vi "Ensure Visible.vi"(10 "Line Numbers":refnum<vi>, 11 "String in":refnum<vi>) -> (2 "Scroll Position":u32, 3 "String out":refnum<vi>)   [LabVIEW 2016, in "Code String.lvclass"]
doc: "Checks the scroll position of <b>String</b> against the selected line in <b>Line Numbers</b> and adjusts the scroll position if the selected line is not range.\nReturns the resulting <b>Scroll Position</b>.\n--------------------\nCopyright (c) 2019 Analog Devices, Inc. All rights reserved.\n\nRedistribution and use in source and binary forms, with or without modification,\nare permitted provided that the following conditions are met:\n - Redistributions of source code must retain the above copyright notice, this\n list of conditions and the following disclaimer.\n - Redistributions in binary form must reproduce the above copyright notice,\n this list of conditions and the following disclaimer in the documentation\n and/or other materials provided with the distribution.\n - Modified versions of the software must be conspicuously marked as such.\n - This software is licensed solely and exclusively for use with\n processors/products manufactured by or for Analog Devices, Inc.\n - This software may not be combined or merged with other code in any manner\n that would cause the software to become subject to terms and conditions\n which differ from those listed here.\n - Neither the name of Analog Devices, Inc. nor the names of its contributors\n may be used to endorse or promote products derived from this software\n without specific prior written permission.\n - The use of this software may or may not infringe the patent rights of one or\n more patent holders. This license does not release you from the requirement\n that you obtain separate licenses from these patent holders to use this\n software.\n\nTHIS SOFTWARE IS PROVIDED BY ANALOG DEVICES, INC. AND CONTRIBUTORS \"AS IS\" AND\nANY EXPRESS OR IMPLIED WARRANTIES, INCLUDING, BUT NOT LIMITED TO,\nNON-INFRINGEMENT, TITLE, MERCHANTABILITY AND FITNESS FOR A PARTICULAR PURPOSE\nARE DISCLAIMED. IN NO EVENT SHALL ANALOG DEVICES, INC. OR CONTRIBUTORS BE LIABLE\nFOR ANY DIRECT, INDIRECT, INCIDENTAL, SPECIAL, EXEMPLARY, PUNITIVE OR\nCONSEQUENTIAL DAMAGES (INCLUDING, BUT NOT LIMITED TO, DAMAGES ARISING OUT OF\nCLAIMS OF INTELLECTUAL PROPERTY RIGHTS INFRINGEMENT; PROCUREMENT OF SUBSTITUTE\nGOODS OR SERVICES; LOSS OF USE, DATA, OR PROFITS; OR BUSINESS INTERRUPTION)\nHOWEVER CAUSED AND ON ANY THEORY OF LIABILITY, WHETHER IN CONTRACT, STRICT\nLIABILITY, OR TORT (INCLUDING NEGLIGENCE OR OTHERWISE) ARISING IN ANY WAY OUT OF\nTHE USE OF THIS SOFTWARE, EVEN IF ADVISED OF THE POSSIBILITY OF SUCH DAMAGE.\n\n2019-01-10-7CBSD SLA"
uses:
  Code String.lvclass
panel:
  # "Copyright (c) 2019 Analog Devices, Inc.  All rights reserved.\n\nRedistribution and use in source and binary forms, with or without modification,\nare permitted provided that the following conditions are met:\n  - Redistributions of source code must retain the above copyright notice, this\n    list of conditions and the following disclaimer.\n  - Redistributions in binary form must reproduce the above copyright notice,\n    this list of conditions and the following disclaimer in the documentation\n    and/or other materials provided with the distribution.\n  - Modified versions of the software must be conspicuously marked as such.\n  - This software is licensed solely and exclusively for use with\n    processors/products manufactured by or for Analog Devices, Inc.\n  - This software may not be combined or merged with other code in any manner\n    that would cause the software to become subject to terms and conditions\n    which differ from those listed here.\n  - Neither the name of Analog Devices, Inc. nor the names of its contributors\n    may be used to endorse or promote products derived from this software\n    without specific prior written permission.\n  - The use of this software may or may not infringe the patent rights of one or\n    more patent holders.  This license does not release you from the requirement\n    that you obtain separate licenses from these patent holders to use this\n    software.\n\nTHIS SOFTWARE IS PROVIDED BY ANALOG DEVICES, INC. AND CONTRIBUTORS \"AS IS\" AND\nANY EXPRESS OR IMPLIED WARRANTIES, INCLUDING, BUT NOT LIMITED TO,\nNON-INFRINGEMENT, TITLE, MERCHANTABILITY AND FITNESS FOR A PARTICULAR PURPOSE\nARE DISCLAIMED. IN NO EVENT SHALL ANALOG DEVICES, INC. OR CONTRIBUTORS BE LIABLE\nFOR ANY DIRECT, INDIRECT, INCIDENTAL, SPECIAL, EXEMPLARY, PUNITIVE OR\nCONSEQUENTIAL DAMAGES (INCLUDING, BUT NOT LIMITED TO, DAMAGES ARISING OUT OF\nCLAIMS OF INTELLECTUAL PROPERTY RIGHTS INFRINGEMENT; PROCUREMENT OF SUBSTITUTE\nGOODS OR SERVICES; LOSS OF USE, DATA, OR PROFITS; OR BUSINESS INTERRUPTION)\nHOWEVER CAUSED AND ON ANY THEORY OF LIABILITY, WHETHER IN CONTRACT, STRICT\nLIABILITY, OR TORT (INCLUDING NEGLIGENCE OR OTHERWISE) ARISING IN ANY WAY OUT OF\nTHE USE OF THIS SOFTWARE, EVEN IF ADVISED OF THE POSSIBILITY OF SUCH DAMAGE.\n\n2019-01-10-7CBSD SLA"
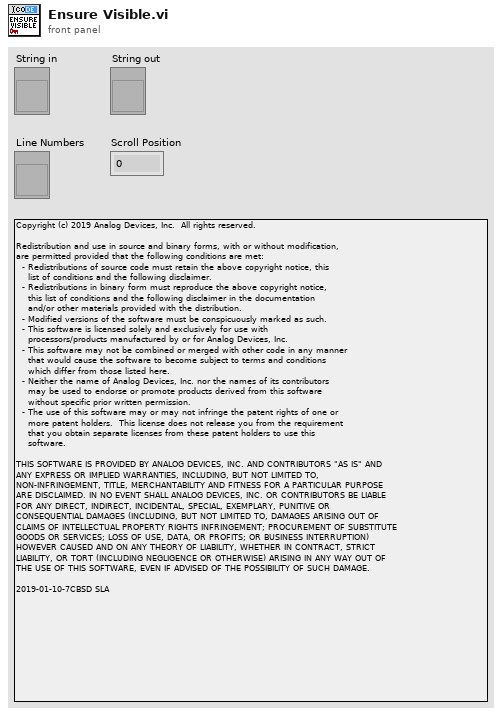
[diagram p1: front panel]
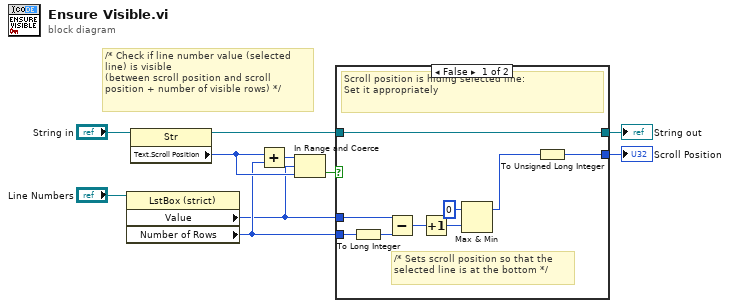
[diagram p0: block diagram]
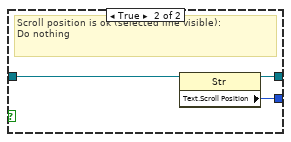
[diagram p2: hidden frame]
diagram:
  # "/* Check if line number value (selected line) is visible\n(between scroll position and scroll position + number of visible rows) */"
  n1 = property on="Property Node" class="LstBox (strict)"(reference="Line Numbers") -> ("Value"=w1:i32, "Number of Rows"=w2:u32)  [unwired: 1 in, 2 out]
  n2 = property on="Property Node" class="Str"(reference="String in") -> (reference out=w5:refnum<vi>, "Text.Scroll Position"=w6:u32)  [unwired: 1 in, 1 out]
  n3 = Add(x=w6, y=w2) -> (x+y=w7:u32)
  n4 = In Range and Coerce(upper limit=w7, x=w1, lower limit=w6) -> (In Range?=w4:bool)  [unwired: 1 out]
  n5 = case shown="False" w4 {
    tunnel: w5 -> [w19 w22]
    tunnel: [w11 w21] -> w8
    tunnel: [w19 w20] -> w3
    tunnel: w2 -> [w15 _]
    tunnel: w1 -> [w14 _]
    frame False {
      # "/* Sets scroll position so that the selected line is at the bottom */"
      # "Scroll position is hiding selected line:\nSet it appropriately"
      n6 = To Long Integer(number=w15) -> (32bit integer=w13:i32)
      n7 = Subtract(x=w14, y=w13) -> (x-y=w16:i32)
      n8 = Increment(x=w16) -> (x+1=w18:i32)
      n9 = Max & Min(x=0, y=w18) -> (max(x,y)=w12:i32)  [unwired: 1 out]
      n10 = To Unsigned Long Integer(number=w12) -> (unsigned 32bit integer=w11:u32)
    }
    frame True {
      # "Scroll position is ok (selected line visible):\nDo nothing"
      n11 = property class="Str"(reference=w22) -> (reference out=w20:refnum<vi>, "Text.Scroll Position"=w21:u32)  [unwired: 1 in, 1 out]
    }
  }
  "Scroll Position" <- w8
  "String out" <- w3
